vi "GetAttributeViReal64_Advanced.vi"(8 "error in (no error)":errorcluster {"code" format="%.0x"}, 9 "AttributeID":u32(ring)=1950003 items=["IVILXISYNC_ARM_ALARM_PERIOD"=1950003, "IVILXISYNC_ARM_ALARM_TIME_FRACTION"=1950005, "IVILXISYNC_ARM_ALARM_TIME_SECONDS"=1950006, "IVILXISYNC_ARM_DELAY"=1950008, "IVILXISYNC_TRIGGER_ALARM_PERIOD"=1950017, "IVILXISYNC_TRIGGER_ALARM_TIME_FRACTION"=1950019, "IVILXISYNC_TRIGGER_ALARM_TIME_SECONDS"=1950020, "IVILXISYNC_TRIGGER_SOURCE_DELAY"=1950024, "MARKER_AMPLITUDE"=1250202, "MARKER_FREQUENCY_COUNTER_RESOLUTION"=1250206, "MARKER_POSITION"=1250207, "MARKER_THRESHOLD"=1250208, "OUTPUT_ARBITRARY_IF"=1150682, "PEAK_EXCURSION"=1250210, "PRESELECTOR_ADJUST"=1150584, "REFERENCE_LEVEL_OFFSET"=1250012, "REFERENCE_LEVEL"=1250011, "REFERENCE_MARKER_AMPLITUDE"=1250801, "REFERENCE_MARKER_POSITION"=1250802, "REFOSCILLATOR_EXTERNAL_FREQUENCY "=1150878, "RESOLUTION_BANDWIDTH"=1250013, "SWEEP_TIME"=1250016, "TRIGGER_AUTO_TIME "=1150844, "TRIGGER_EXTERNAL2_DELAY"=1150669, "TRIGGER_EXTERNAL2_LEVEL"=1150670, "TRIGGER_EXTERNAL_DELAY"=1150668, "TRIGGER_EXTERNAL_LEVEL"=1150802, "TRIGGER_FRAME_DELAY "=1150842, "TRIGGER_FRAME_OFFSET "=1150840, "TRIGGER_FRAME_PERIOD "=1150839, "TRIGGER_HOLD_OFF_TIME "=1150847, "TRIGGER_LINE_DELAY"=1150837, "TRIGGER_RFBURST_DELAY"=1150831, "TRIGGER_RFBURST_LEVEL_RELATIVE"=1150829, "TRIGGER_RFBURST_TRIGGER_RFBURST_LEVEL_ABSOLUTE "=1150828, "TRIGGER_VIDEO_DELAY"=1150672, "TRIGGER_VIDEO_LEVEL"=1150805, "UNITS_PER_DIVISION"=1250601, "VIDEO_BANDWIDTH"=1250022, "VIDEO_TRIGGER_LEVEL"=1250501], 10 "RepCapIdentifier":string, 11 "instrument handle":refnum<k15>) -> (0 "error out":errorcluster {"code" format="%.0x"}, 2 "AttributeValue":dbl, 3 "instrument handle out":refnum<k15>)   [LabVIEW 2009, in "Keysight XSAn.lvlib"]
doc: "Gets a Real64 attribute from the instrument driver.\nThe following Attributes are supported:\n\nIVILXISYNC_ARM_ALARM_PERIOD\nIVILXISYNC_ARM_ALARM_TIME_FRACTION\nIVILXISYNC_ARM_ALARM_TIME_SECONDS\nIVILXISYNC_ARM_DELAY\nIVILXISYNC_TRIGGER_ALARM_PERIOD\nIVILXISYNC_TRIGGER_ALARM_TIME_FRACTION\nIVILXISYNC_TRIGGER_ALARM_TIME_SECONDS\nIVILXISYNC_TRIGGER_SOURCE_DELAY\nMARKER_AMPLITUDE\nMARKER_FREQUENCY_COUNTER_RESOLUTION\nMARKER_POSITION\nMARKER_THRESHOLD\nOUTPUT_ARBITRARY_IF\nPEAK_EXCURSION\nPRESELECTOR_ADJUST\nREFERENCE_LEVEL_OFFSET\nREFERENCE_LEVEL\nREFERENCE_MARKER_AMPLITUDE\nREFERENCE_MARKER_POSITION\nREFOSCILLATOR_EXTERNAL_FREQUENCY \nRESOLUTION_BANDWIDTH\nSWEEP_TIME\nTRIGGER_AUTO_TIME\nTRIGGER_EXTERNAL2_DELAY\nTRIGGER_EXTERNAL2_LEVEL\nTRIGGER_EXTERNAL_DELAY\nTRIGGER_EXTERNAL_LEVEL\nTRIGGER_FRAME_DELAY\nTRIGGER_FRAME_OFFSET\nTRIGGER_FRAME_PERIOD\nTRIGGER_HOLD_OFF_TIME\nTRIGGER_LINE_DELAY\nTRIGGER_RFBURST_DELAY\nTRIGGER_RFBURST_LEVEL_RELATIVE\nTRIGGER_RFBURST_TRIGGER_RFBURST_LEVEL_ABSOLUTE\nTRIGGER_VIDEO_DELAY\nTRIGGER_VIDEO_LEVEL \nUNITS_PER_DIVISION\nVIDEO_BANDWIDTH\nVIDEO_TRIGGER_LEVEL"
uses:
  <instrlib>/Keysight XSAn/Keysight XSAn.lvlib
  AgXSAn.dll
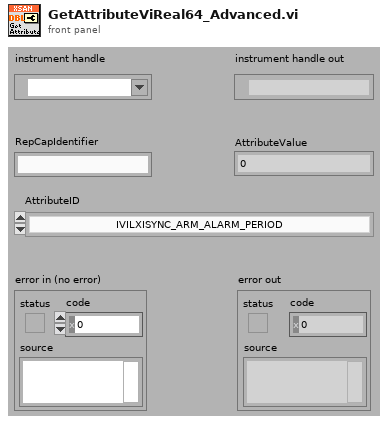
[diagram p1: front panel]
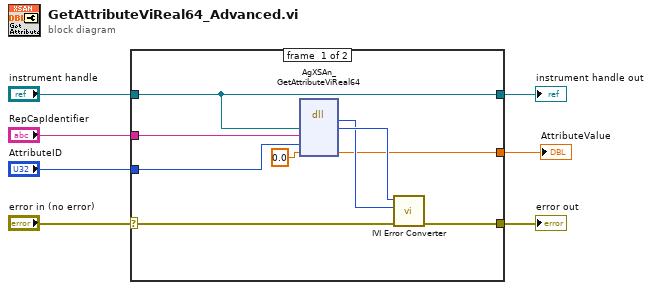
[diagram p0: block diagram]
diagram:
  n1 = case shown="No Error" "error in (no error)" {
    selector: "error in (no error)" -> [w14 w18]
    tunnel: [w13 w18] -> w7
    tunnel: "instrument handle" -> [w8 w17]
    tunnel: "RepCapIdentifier" -> [w12 _]
    tunnel: "AttributeID" -> [w11 _]
    tunnel: [w9 _] -> w2
    tunnel: [w8 w17] -> w1
    frame #0 {
      n2 = dll-call lib="AgXSAn**.dll" fn="AgXSAn_GetAttributeViReal64"("Vi"=w8, "RepCapIdentifier"=w12, "AttributeID"=w11, "AttributeValue"=0.0) -> ("return type"=w15:i32, "Vi"=w16:u32, "AttributeValue"=w9:dbl)  [unwired: 5 in, 2 out]
      n3 = call <instrlib>:"IVI Error Converter.vi"("error in (no error)"=w14, "IVI error code (0)"=w15, "instrument handle"=w16) -> ("error out"=w13:errorcluster)  [unwired: 7 in, 1 out]
    }
    frame #1 {
    }
  }
  "error out" <- w7
  "instrument handle out" <- w1
  "AttributeValue" <- w2
